vi "Build Minor Frames.vi"(8 "error in (no error)":errorcluster, 11 "Bus Controller XML Node":refnum<k20>) -> (0 "error out":errorcluster, 3 "Minor Frames":refnum<class "Minor Frame.lvclass">[](array[class]))   [LabVIEW 2020]
doc: "Retrieves all the Minor Frame nodes defined in the XML. All Messages contained in the Minor Frames then have their names retrieved and stored in ordr as the Minor Frame sequence. The Messages should all have unique names."
uses:
  Frames & Messages/Minor Frame/Minor Frame.lvclass
  <vilib>/xml/NI_XML.lvlib
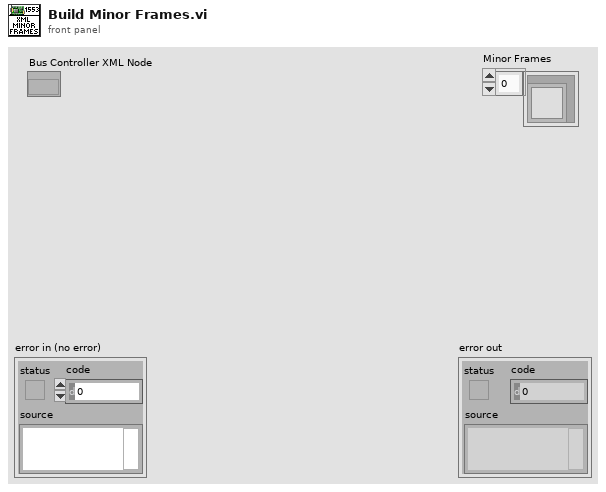
[diagram p1: front panel]
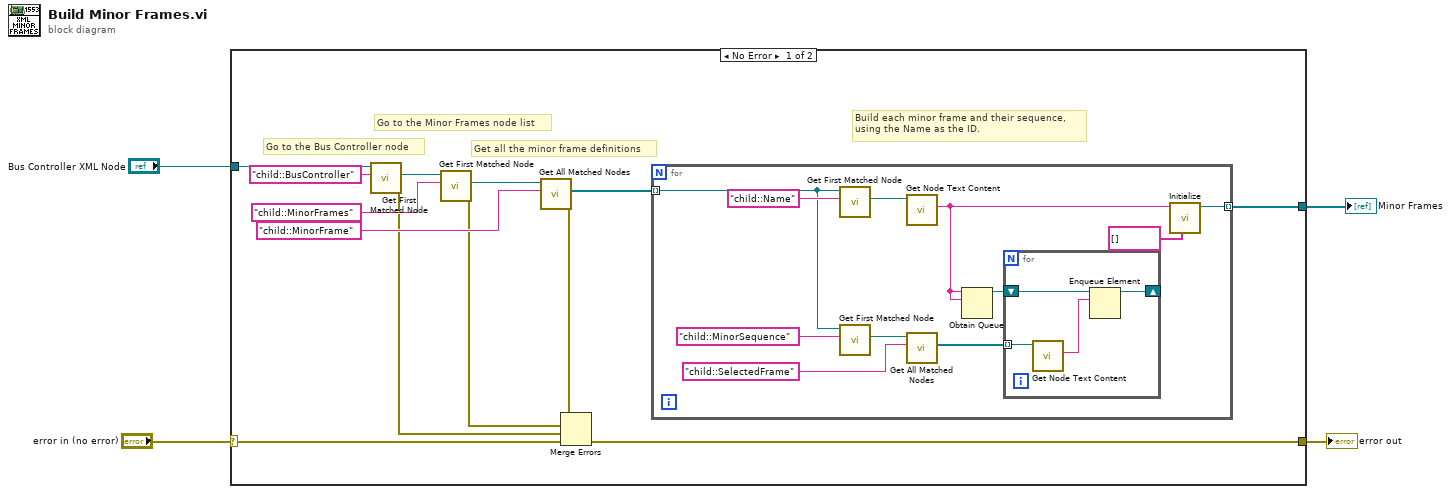
[diagram p0: block diagram]
diagram:
  n1 = case shown="No Error" "error in (no error)" {
    selector: "error in (no error)" -> [w9 w33]
    tunnel: [w8 w33] -> w3
    tunnel: "Bus Controller XML Node" -> [w17 _]
    tunnel: [w10 _] -> w1
    frame No Error {
      # "Build each minor frame and their sequence,\nusing the Name as the ID."
      # "Get all the minor frame definitions"
      # "Go to the Minor Frames node list"
      # "Go to the Bus Controller node"
      n2 = call <vilib>:"Get First Matched Node.vi"("XPath expression"="child::BusController", "node in"=w17) -> ("error out"=w7:errorcluster, "node result"=w15:refnum<k20>)  [unwired: 7 in, 1 out]
      n3 = call <vilib>:"Get First Matched Node.vi"("XPath expression"="child::MinorFrames", "node in"=w15) -> ("error out"=w6:errorcluster, "node result"=w13:refnum<k20>)  [unwired: 7 in, 1 out]
      n4 = call <vilib>:"Get All Matched Nodes.vi"("XPath expression"="child::MinorFrame", "node in"=w13) -> ("error out"=w5:errorcluster, "node result array"=w11:refnum<k20>[])  [unwired: 7 in, 1 out]
      n5 = Merge Errors(w5, w6, w7, w9) -> (w8:errorcluster)
      n6 = for {
        tunnel: w11 -> [w26] mode=indexing
        tunnel: [w24] -> w10 mode=indexing
        n7 = call <vilib>:"Get First Matched Node.vi"("XPath expression"="child::Name", "node in"=w26) -> ("node result"=w27:refnum<k20>)  [unwired: 7 in, 2 out]
        n8 = call <vilib>:"Get First Matched Node.vi"("XPath expression"="child::MinorSequence", "node in"=w26) -> ("node result"=w22:refnum<k20>)  [unwired: 7 in, 2 out]
        n9 = call <vilib>:"Get Node Text Content.vi"("node in"=w27) -> ("node text"=w19:string)  [unwired: 8 in, 2 out]
        n10 = call <vilib>:"Get All Matched Nodes.vi"("XPath expression"="child::SelectedFrame", "node in"=w22) -> ("node result array"=w21:refnum<k20>[])  [unwired: 7 in, 2 out]
        n11 = Obtain Queue(name (unnamed)=w19, element data type=w19) -> (queue out=w20:refnum<queue>)  [unwired: 3 in, 2 out]
        n12 = for {
          tunnel: w21 -> [w32] mode=indexing
          shift-right: [w29] -> _
          shift-left: w20 -> [w31]
          n13 = call <vilib>:"Get Node Text Content.vi"("node in"=w32) -> ("node text"=w30:string)  [unwired: 8 in, 2 out]
          n14 = Enqueue Element(queue=w31, element=w30) -> (queue out=w29:refnum<queue>)  [unwired: 2 in, 2 out]
        }
        n15 = call "Initialize.vi"("Schedule"=string[] [], "ID"=w19) -> ("Minor Frame out"=w24:refnum<class "Minor Frame.lvclass">)  [unwired: 8 in, 1 out]
      }
    }
    frame Error {
    }
  }
  "error out" <- w3
  "Minor Frames" <- w1
